vi "G-Audio Capture Example (LINX).vi"() -> ()   [LabVIEW 2020]
doc: "Simple example of audio device capture, saving the acquired data to a WAV file."
uses:
  <vilib>/Dataflow_G/G-Audio/Controls/Audio Device Info.ctl
  <vilib>/Dataflow_G/G-Audio/Controls/Audio Device Type.ctl
  <vilib>/Dataflow_G/G-Audio/Controls/Audio Device Native Data Format.ctl
  <vilib>/Dataflow_G/G-Audio/Controls/Audio Device Format.ctl
  <vilib>/Dataflow_G/G-Audio/Controls/Audio Device Config.ctl
  d37775a1-27ef-4781-ba3e-b38a0bb78134.vi
  <vilib>/Dataflow_G/G-Audio/Private/Result To Error.vi
  d37775a1-27ef-4781-ba3e-b38a0bb78134.vi/6b901882-6109-4f44-aca5-48e1525e5248.vi
  d37775a1-27ef-4781-ba3e-b38a0bb78134.vi/06c0137a-63d3-4e30-982f-115d83a1188c.vi
  <vilib>/Dataflow_G/G-Audio/Audio Devices/Get Audio Device Configuration.vi
  <vilib>/Dataflow_G/G-Audio/Private/Audio Device Refnum To Value.vi
  d37775a1-27ef-4781-ba3e-b38a0bb78134.vi/06c0137a-63d3-4e30-982f-115d83a1188c.vi/4b7b629c-2e91-4160-9820-a26af8f6e677.vi
  <vilib>/Dataflow_G/G-Audio/Private/ma_format To Audio Data Format.vi
  <vilib>/Utility/Data Type/Get Numeric Information.vi
  <vilib>/Utility/error.llb/Error Cluster From Error Code.vi
  <vilib>/Dataflow_G/G-Audio/G-Audio.lvlib
panel:
  in  "Begin":bool
  out "Capture Devices":T1[](array[typedef])
  out "error out":errorcluster
  in  "Stop":bool
  out "Waveform":waveform(i16)[](graph)
  # "Instructions:\n1. Run the VI.\n2. Select the Capture Device using the array index, then press Being Capture.\n2. The VI will begin audio capture and display the data in the waveform graph.\n3. Press Stop to finish audio capture."
  # "G"
  # "-Audio"
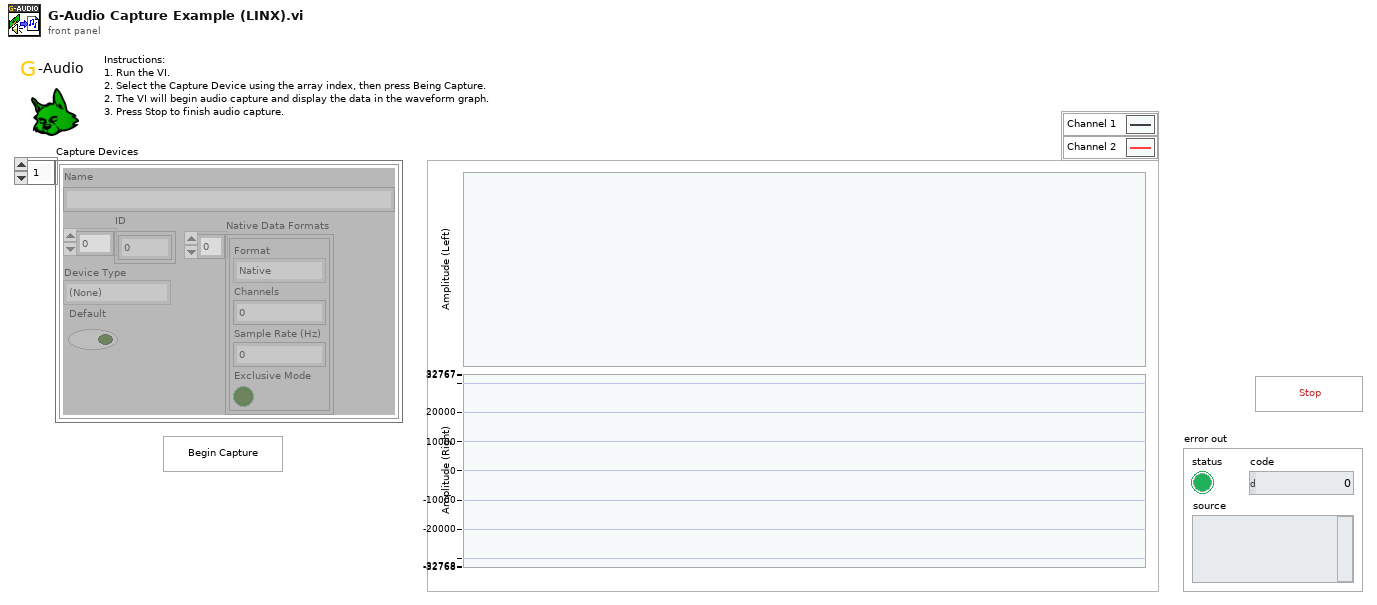
[diagram p1: front panel]
types:
  T1 = typedef "G-Audio.lvlib/Audio Device Info.ctl" = cluster{"Name":string, "ID":u8[], "Device Type":T2, "Default":bool, "Native Data Formats":T3[]}
  T2 = typedef "G-Audio.lvlib/Audio Device Type.ctl" = enum16{"(None)", "Playback", "Capture", "Duplex", "Loopback"}
  T3 = typedef "G-Audio.lvlib/Audio Device Native Data Format.ctl" = cluster{"Format":T4, "Channels":u32, "Sample Rate (Hz)":u32, "Exclusive Mode":bool}
  T4 = typedef "G-Audio.lvlib/Audio Device Format.ctl" = enum16{"Native", "U8", "I16", "I32", "SGL"}
  T5 = typedef "G-Audio.lvlib/Audio Device Config.ctl" = cluster{"Sample Rate (Hz)":u32, "Channels":u32, "Format":T4}
  T6 = typedef "G-Audio.lvlib/Audio Device Refnum.ctl" = refnum<file>
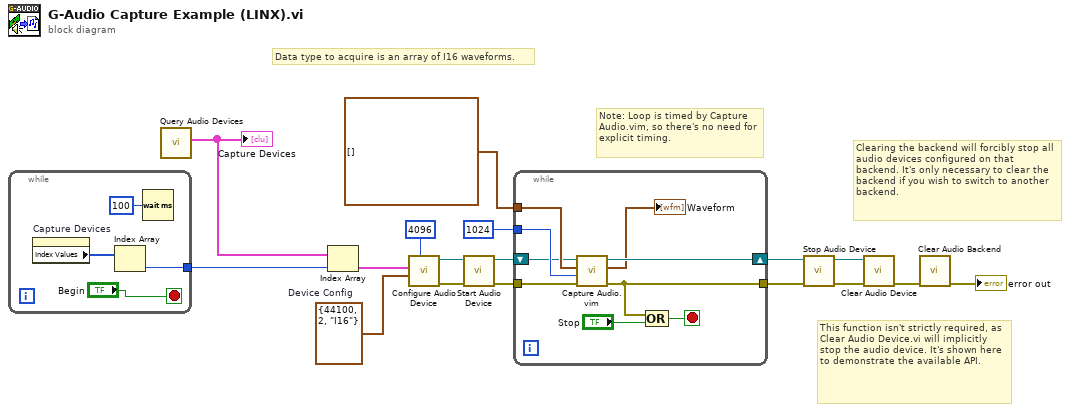
[diagram p0: block diagram]
diagram:
  w8 = T5 {"Sample Rate (Hz)"=44100, "Channels"=2, "Format"=enum."I16"}  # Device Config
  # "Data type to acquire is an array of I16 waveforms."
  # "This function isn't strictly required, as Clear Audio Device.vi will implicitly stop the audio device. It's shown here to demonstrate the available API."
  # "Clearing the backend will forcibly stop all audio devices configured on that backend. It's only necessary to clear the backend if you wish to switch to another backend."
  # "Note: Loop is timed by Capture Audio.vim, so there's no need for explicit timing."
  n1 = while {
    tunnel: [w20] -> w1
    stop <- "Begin" stop-if-true
    n2 = property on="Capture Devices" class="Arr (strict)"() -> ("Index Values"=w21:u32[])  [unwired: 2 in, 2 out]
    n3 = Index Array(array=w21) -> (element=w20:u32)  [unwired: 1 in]
    n4 = Wait (ms)(milliseconds to wait=u32 100) -> ()  [unwired: 1 out]
  }
  n5 = call <vilib>:"Query Audio Devices.vi"() -> ("Capture Devices"=w3:T1[])  [unwired: 7 in, 4 out]
  "Capture Devices" <- w3
  n6 = Index Array(array=w3, index=w1) -> (element=w2:T1)
  n7 = call <vilib>:"Configure Audio Device.vi"("Buffer Size (4096)"=4096 ("number of samples/ch"), "Device Config"=w8, "Audio Device"=w2) -> ("error out"=w11:errorcluster, "Audio Device Refnum"=w10:T6)  [unwired: 5 in, 2 out]
  n8 = call <vilib>:"Start Audio Device.vi"("error in (no error)"=w11, "Audio Device Refnum In"=w10) -> ("error out"=w14:errorcluster, "Audio Device Refnum Out"=w15:T6)  [unwired: 8 in]
  n9 = while {
    shift-right: [w30] -> w6
    shift-left: w15 -> [w23]
    tunnel: w14 -> [w22]
    tunnel: 1024 ("number of samples/ch") -> [w27]
    tunnel: waveform(i16)[] [] -> [w26]
    tunnel: [w24] -> w4
    stop <- w29 stop-if-true
    n10 = call "Capture Audio.vim"("error in (no error)"=w22, "Samples To Read"=w27, "Data Format"=w26, "Audio Device Refnum In"=w23) -> ("error out"=w24:errorcluster, "Audio Data"=→"Waveform":waveform(i16)[], "Audio Device Refnum Out"=w30:T6)  [unwired: 5 in]
    n11 = Compound Arithmetic op=OR(w24, "Stop") -> (w29:bool)
  }
  n12 = call <vilib>:"Stop Audio Device.vi"("error in (no error)"=w4, "Audio Device Refnum In"=w6) -> ("error out"=w16:errorcluster, "Audio Device Refnum Out"=w17:T6)  [unwired: 8 in]
  n13 = call <vilib>:"Clear Audio Device.vi"("error in (no error)"=w16, "Audio Device Refnum In"=w17) -> ("error out"=w13:errorcluster)  [unwired: 9 in]
  n14 = call <vilib>:"Clear Audio Backend.vi"("error in (no error)"=w13) -> ("error out"=→"error out":errorcluster)  [unwired: 10 in]
